vi "Post-Build Action.vi"(5 "Files Generated by Build":path[](array[path]), 6 "Top Level/Always Included VIs":path[](array[path]), 7 "Destination Path":path, 8 "error in (no error)":errorcluster, 9 "Target Name":string, 10 "Build Specification Name":string, 11 "Project Path":path) -> (0 "error out":errorcluster)   [LabVIEW 2021]
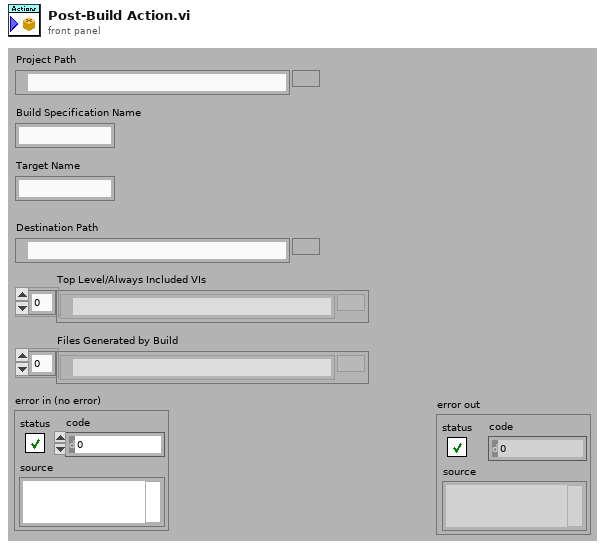
[diagram p1: front panel]
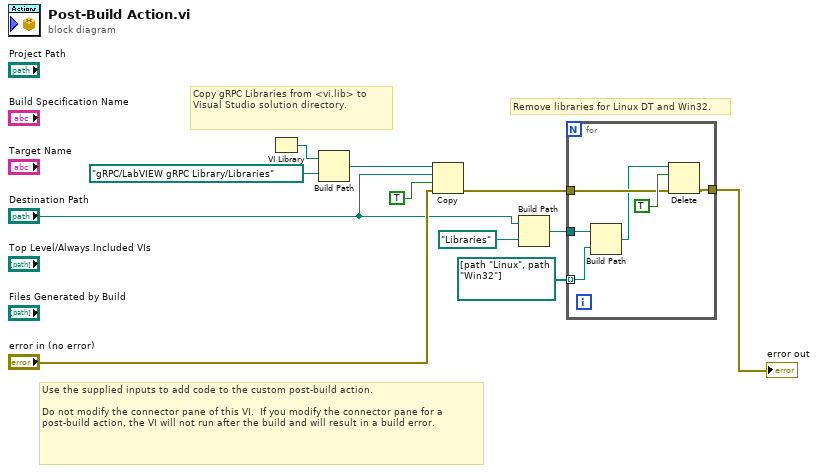
[diagram p0: block diagram]
diagram:
  # "Remove libraries for Linux DT and Win32."
  # "Copy gRPC Libraries from <vi.lib> to Visual Studio solution directory."
  # "Use the supplied inputs to add code to the custom post-build action.\n\nDo not modify the connector pane of this VI.  If you modify the connector pane for a post-build action, the VI will not run after the build and will result in a build error."
  n1 = VI Library() -> (path=w11:path)
  n2 = Build Path(base path=w11, name or relative path=path "gRPC/LabVIEW gRPC Library/Libraries" ("path")) -> (appended path=w9:path)
  n3 = Copy(8:"error in (no error)", 9:TRUE ("overwrite (F)"), 10:"Destination Path", 11:w9) -> (0:w4:errorcluster)  [unwired: 1 in, 2 out]
  n4 = Build Path(base path="Destination Path", name or relative path=path "Libraries" ("path")) -> (appended path=w3:path)
  n5 = for {
    tunnel: w4 -> [w16]
    tunnel: w3 -> [w15]
    tunnel: path[] [path "Linux", path "Win32"] -> [w14] mode=indexing
    tunnel: [w12] -> w1
    n6 = Build Path(base path=w15, name or relative path=w14) -> (appended path=w13:path)
    n7 = Delete(path (use dialog)=w13, entire hierarchy (F)=TRUE, error in=w16) -> (error out=w12:errorcluster)  [unwired: 2 in, 2 out]
  }
  "error out" <- w1
